vi "SerialPort.vi"(1 "SerialSettings":T1={"SerialPort"="RS232\\Port1", "TxFIFO"="U64FIFOTx", "RxFIFO"="U64FIFORx", "TimestampRegister"="TimestampRegister"}) -> ()   [LabVIEW 2016, in "FPGASerial.lvlib"]
uses:
  FPGASerial.lvlib
  DataTypes/SerialSettings.ctl
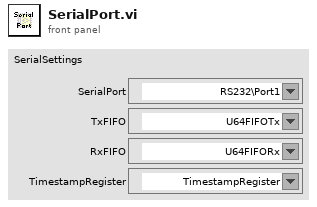
[diagram p1: front panel]
types:
  T1 = typedef "FPGASerial.lvlib/SerialSettings.ctl" = cluster{"SerialPort":refnum<k21>, "TxFIFO":refnum<k21>, "RxFIFO":refnum<k21>, "TimestampRegister":refnum<k21>}
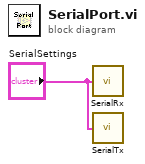
[diagram p0: block diagram]
diagram:
  n1 = call "SerialRx.vi"("SerialSettings"="SerialSettings") -> ()  [unwired: 1 in]
  n2 = call "SerialTx.vi"("SerialSettings"="SerialSettings") -> ()  [unwired: 1 in]
